vi "teststringconcatation.vi"() -> ()   [LabVIEW 2012]
panel:
  in  "Enum":enum16{"foo", "bar", "baz", ""}(ring)
  out "concatenated string":string
  in  "stop":bool
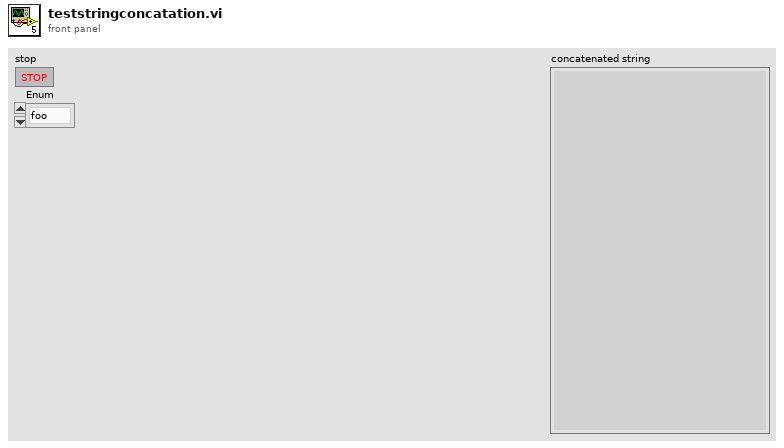
[diagram p1: front panel]
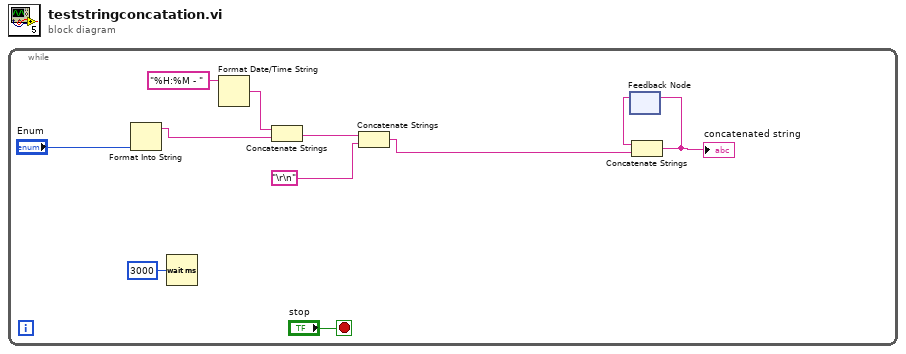
[diagram p0: block diagram]
diagram:
  n1 = while {
    stop <- "stop" stop-if-true
    n2 = Format Into String("Enum") -> (resulting string=w4:string)  [unwired: 3 in, 1 out]
    n3 = Wait (ms)(milliseconds to wait=u32 3000) -> ()  [unwired: 1 out]
    n4 = Format Date/Time String(time format string (%c)="%H:%M - ") -> (date/time string=w5:string)  [unwired: 2 in]
    n5 = Concatenate Strings(w5, w4) -> (w3:string)
    n6 = Concatenate Strings(w3, "\r\n") -> (w1:string)
    n7 = feedback #1() -> (w7:string)  [unwired: 1 in]
    n8 = Concatenate Strings(w7, w1) -> (w8:string)
    "concatenated string" <- w8
    n9 = feedback-in #1(w8) -> ()
  }
